vi "Update Chart Selection.vi"(8 "error in (no error)":errorcluster, 10 "Chart Selection":T1, 11 "Historian Charting Manager in":refnum<class "Historian Charting Manager.lvclass">) -> (0 "error out":errorcluster, 3 "Historian Charting Manager out":refnum<class "Historian Charting Manager.lvclass">)   [LabVIEW 2020, in "VolatusGUI.lvlib" / "Historian Charting Manager.lvclass"]
uses:
  Historian Charting Manager.lvclass
  Historian Charting Manager.lvclass/Historian Charting Manager.ctl
  Chart Selection.ctl
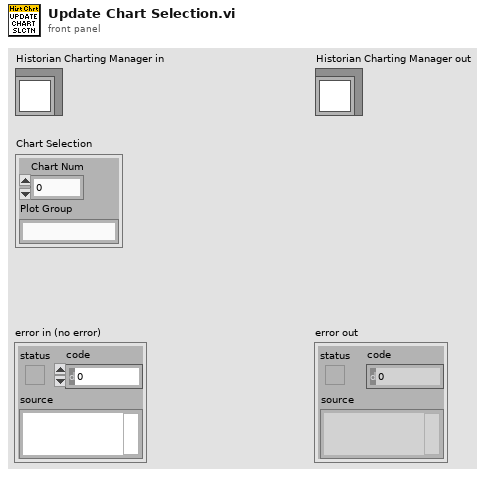
[diagram p1: front panel]
types:
  T1 = typedef "VolatusGUI.lvlib/Historian Charting Manager.lvclass/Chart Selection.ctl" = cluster{"Chart Num":i32, "Plot Group":string}
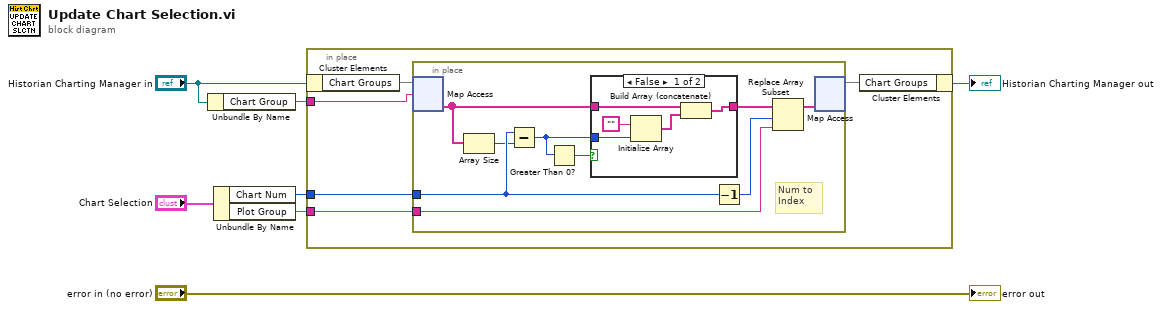
[diagram p0: block diagram]
diagram:
  n1 = Unbundle By Name("Historian Charting Manager in") -> ("Chart Group"=w4:string)
  n2 = Unbundle By Name("Chart Selection") -> ("Chart Num"=w2:i32, "Plot Group"=w1:string)
  n3 = in-place {
    in-place-border: w4 -> [w11]
    in-place-border: w2 -> [w9]
    in-place-border: w1 -> [w8]
    n4 = in-place-cluster #1("Historian Charting Manager in") -> ("Chart Groups"=w12:map{string, string[]})
    n5 = in-place {
      in-place-border: w9 -> [w19]
      in-place-border: w8 -> [w13]
      # "Num to Index"
      n6 = in-place-map #2(w12, w11) -> (w16:string[])  [unwired: 1 in, 1 out]
      n7 = Array Size(array=w16) -> (size(s)=w18:i32)
      n8 = Subtract(x=w19, y=w18) -> (x-y=w14:i32)
      n9 = Greater Than 0?(x=w14) -> (x > 0?=w17:bool)
      n10 = case shown="False" w17 {
        tunnel: w16 -> [w24 w27]
        tunnel: [w23 w27] -> w15
        tunnel: w14 -> [w26 _]
        frame False {
          n11 = Initialize Array("", w26) -> (w22:string[])
          n12 = Build Array (concatenate)(w24, w22) -> (w23:string[])
        }
        frame True {
        }
      }
      n13 = Decrement(x=w19) -> (x-1=w20:i32)
      n14 = Replace Array Subset(array=w15, new element=w13, index=w20) -> (w21:string[])
      n15 = in-place-map #2(w21) -> (w10:map{string, string[]})  [unwired: 1 in, 2 out]
    }
    n16 = in-place-cluster #1("Chart Groups"=w10) -> (→"Historian Charting Manager out":refnum<class "Historian Charting Manager.lvclass">)
  }
  "error out" <- "error in (no error)"
